vi "dfd_Signed WL to Upper Lower Limit.vi"(10 "wl":i16) -> (1 "lower limit":i32, 2 "upper limit":i32)   [LabVIEW 2017, in "NI_DigFilterLicensed.lvlib"]
uses:
  <vilib>/addons/Digital Filter Design/NI_DigFilterLicensed.lvlib
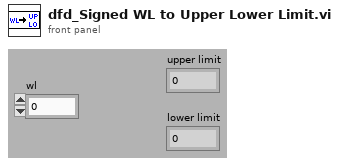
[diagram p1: front panel]
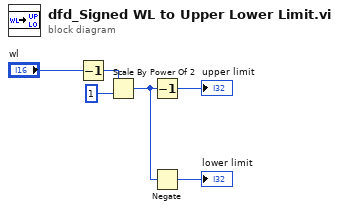
[diagram p0: block diagram]
diagram:
  n1 = Decrement(x="wl") -> (x-1=w5:i16)
  n2 = Scale By Power Of 2(n=w5, x=1) -> (x*2^n=w3:i32)
  n3 = Decrement(x=w3) -> (x-1=→"upper limit":i32)
  n4 = Negate(x=w3) -> (-x=→"lower limit":i32)
